vi "DotNET XML Validate Signature.vi"(8 "error in (no error)":errorcluster, 10 "Signed XML":string) -> (0 "error out":errorcluster, 2 "CheckSignature":bool)   [LabVIEW 2016]
uses:
  System.Xml
  System.Security
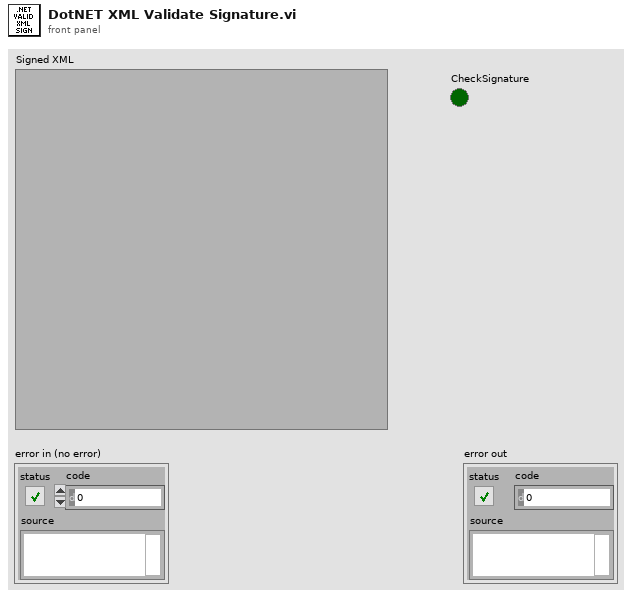
[diagram p1: front panel]
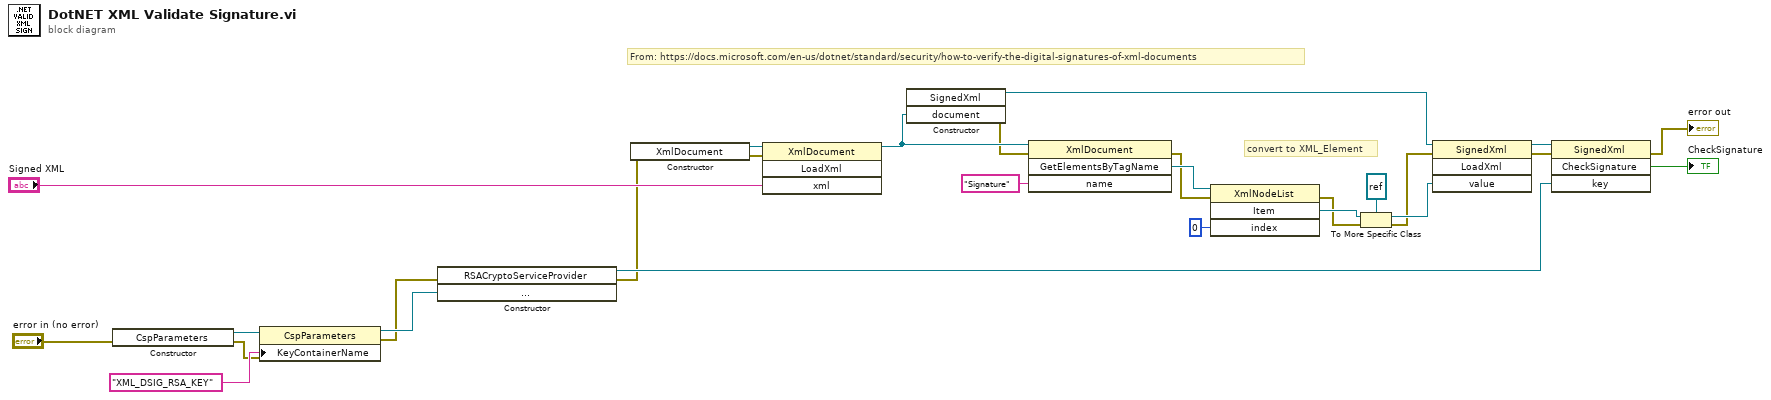
[diagram p0: block diagram]
diagram:
  # "convert to XML_Element"
  # "From: https://docs.microsoft.com/en-us/dotnet/standard/security/how-to-verify-the-digital-signatures-of-xml-documents"
  n1 = constructor class="CspParameters" ("AliceErstelltPrivateKeyUndPublicKey")(error in="error in (no error)") -> (reference out=w27:refnum<k24>, error out=w24:errorcluster)  [unwired: 2 in, 1 out]
  n2 = property class="CspParameters"(reference=w27, error in=w24, "KeyContainerName"="XML_DSIG_RSA_KEY") -> (reference out=w25:refnum<k24>, error out=w23:errorcluster)
  n3 = constructor class="RSACryptoServiceProvider" ("AliceErstelltPrivateKeyUndPublicKey")(error in=w23, "parameters"=w25) -> (reference out=w10:refnum<k24>, error out=w7:errorcluster)  [unwired: 2 in, 2 out]
  n4 = constructor class="XmlDocument"(error in=w7) -> (reference out=w22:refnum<k24>, error out=w21:errorcluster)  [unwired: 2 in, 1 out]
  n5 = invoke class="XmlDocument" method="LoadXml"(reference=w22, error in=w21, "xml"="Signed XML") -> (reference out=w19:refnum<k24>)  [unwired: 1 in, 3 out]
  n6 = constructor class="SignedXml"("document"=w19) -> (reference out=w17:refnum<k24>, error out=w3:errorcluster)  [unwired: 3 in, 2 out]
  n7 = invoke class="XmlDocument" method="GetElementsByTagName"(reference=w19, error in=w3, "name"="Signature") -> (error out=w5:errorcluster, "GetElementsByTagName"=w16:refnum<k24>)  [unwired: 1 in, 2 out]
  n8 = invoke class="XmlNodeList" method="Item"(reference=w16, error in=w5, "index"=0) -> (error out=w4:errorcluster, "Item"=w14:refnum<k24>)  [unwired: 1 in, 2 out]
  n9 = To More Specific Class(target class=refnum<k24> refnum ("reference out"), reference=w14, error in=w4) -> (specific class reference=w12:refnum<k24>, error out=w2:errorcluster)
  n10 = invoke class="SignedXml" method="LoadXml"(reference=w17, error in=w2, "value"=w12) -> (reference out=w11:refnum<k24>, error out=w6:errorcluster)  [unwired: 1 in, 2 out]
  n11 = invoke class="SignedXml" method="CheckSignature"(reference=w11, error in=w6, "key"=w10) -> (error out=→"error out":errorcluster, "CheckSignature"=→"CheckSignature":bool)  [unwired: 1 in, 2 out]
